vi "Parse Algorithm Inputs.vi"(8 "error in (no error)":errorcluster, 11 "Algorithm Information":T2) -> (0 "error out":errorcluster, 1 "Required Q as string":string, 2 "Optional Q as string":string, 3 "Groups of Alternatives":cluster{T1[], "is Optional?":bool}[](array[cluster]), 4 "Q descriptions":string)   [LabVIEW 2013, in "QWTBLVLib.lvlib"]
doc: "Returns parsed informations about required, alternative and parameter input quantities."
uses:
  QWTBLVLib.lvlib
  TD Algorithm Information.ctl
  TD Algorithm Information Input.ctl
  TD Algorithm Information Output.ctl
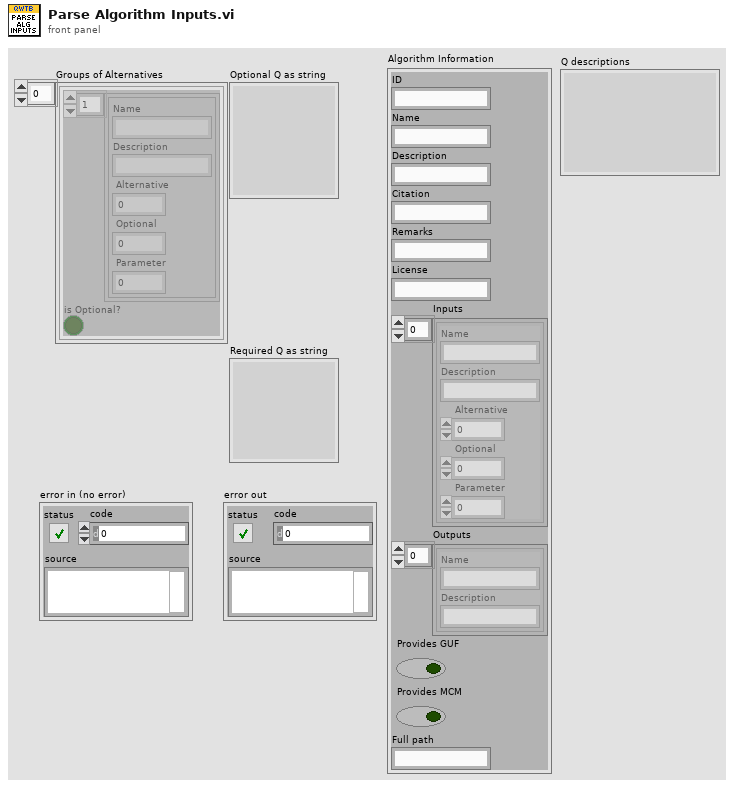
[diagram p1: front panel]
types:
  T1 = typedef "QWTBLVLib.lvlib/TD Algorithm Information Input.ctl" = cluster{"Name":string, "Description":string, "Alternative":i32, "Optional":i32, "Parameter":i32}
  T2 = typedef "QWTBLVLib.lvlib/TD Algorithm Information.ctl" = cluster{"ID":string, "Name":string, "Description":string, "Citation":string, "Remarks":string, "License":string, "Inputs":T1[], "Outputs":T3[], "Provides GUF":bool, "Provides MCM":bool, "Full path":string}
  T3 = typedef "QWTBLVLib.lvlib/TD Algorithm Information Output.ctl" = cluster{"Name":string, "Description":string}
  T4 = cluster{"Group of Alternatives":T1[], "is Group Optional?":bool}[]
  T5 = cluster{"Group of Alternatives":T1[], "is Group Optional?":bool}
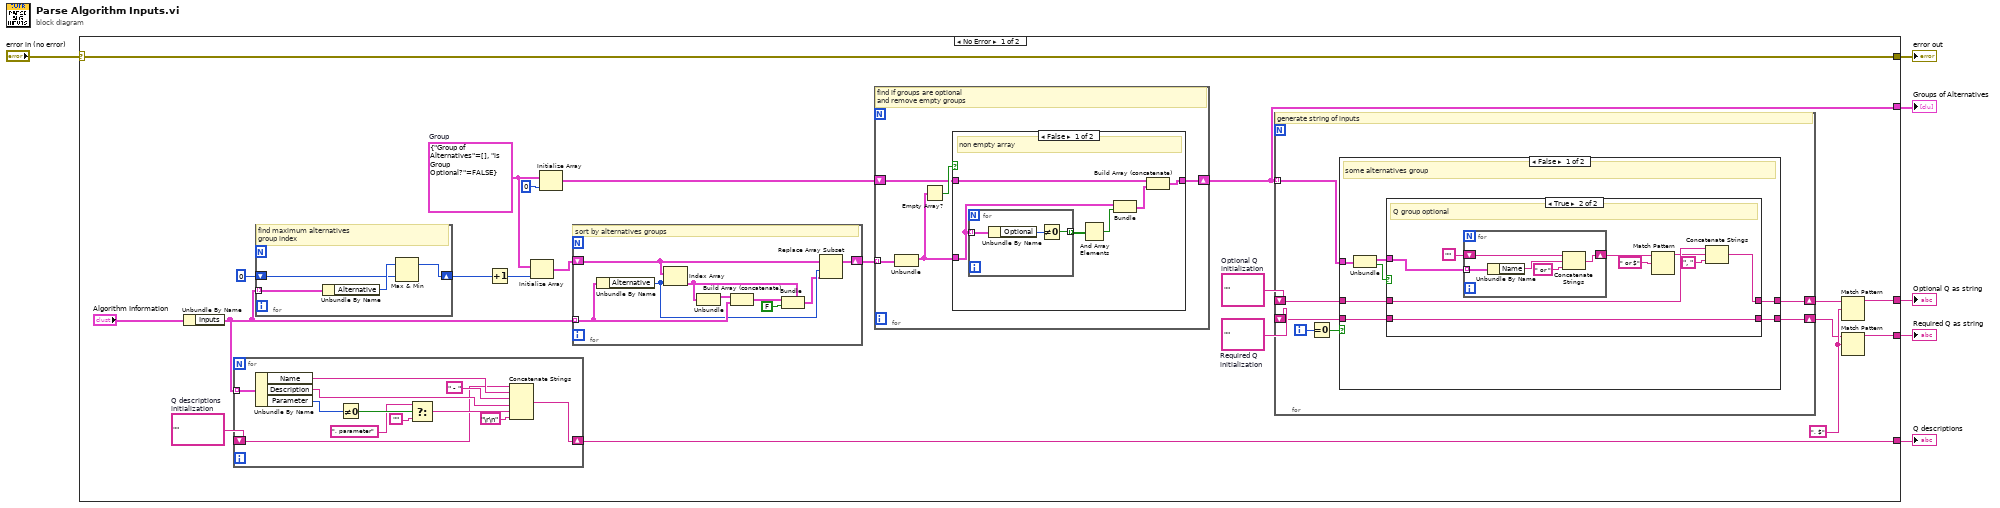
[diagram p0: block diagram]
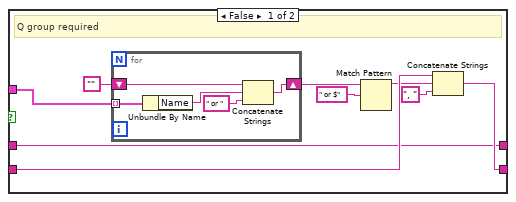
[diagram p2: hidden frame]
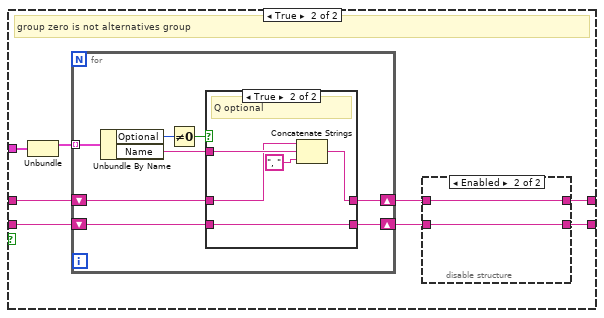
[diagram p3: hidden frame]
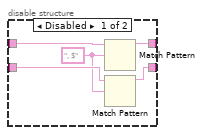
[diagram p4: hidden frame]
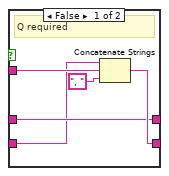
[diagram p5: hidden frame]
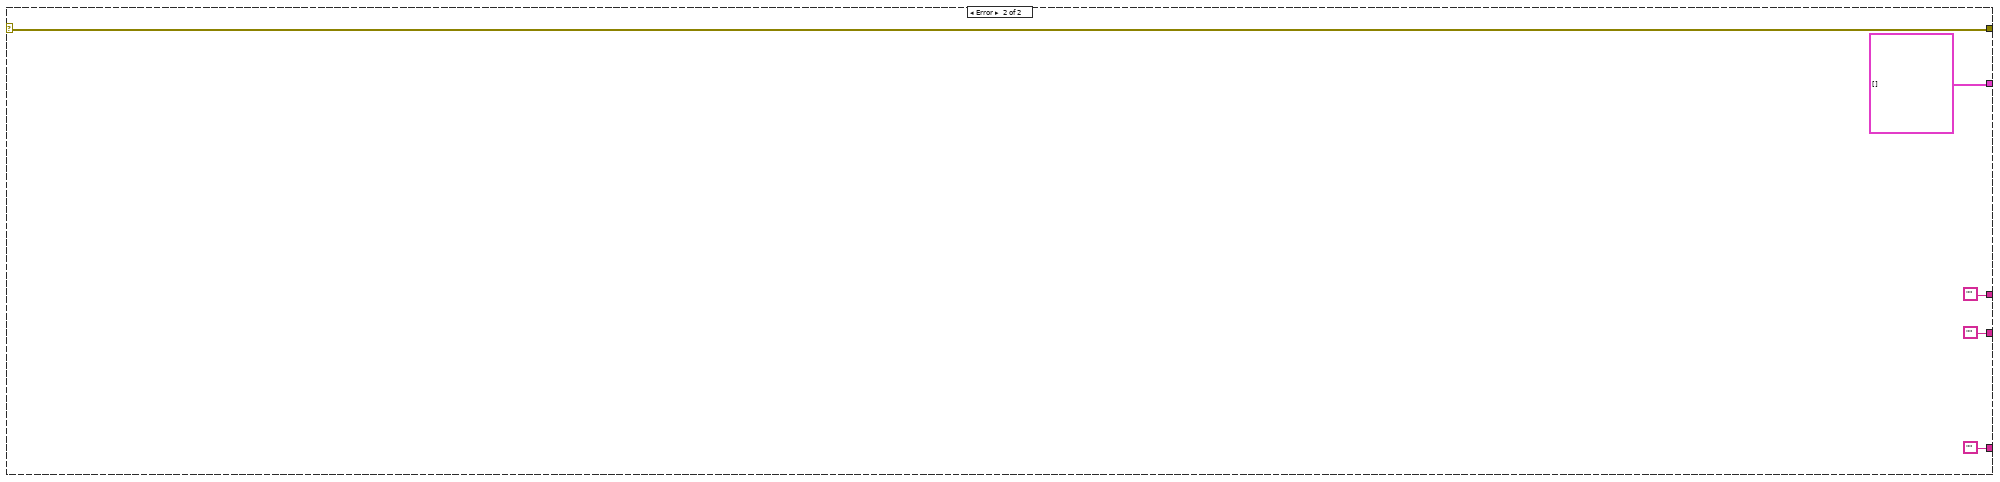
[diagram p7: hidden frame]
diagram:
  n1 = case shown="No Error" "error in (no error)" {
    selector: "error in (no error)" -> [w26 w147]
    tunnel: [w26 w147] -> w6
    tunnel: [w12 T4 []] -> w4
    tunnel: [w9 ""] -> w3
    tunnel: [w8 ""] -> w2
    tunnel: [w7 ""] -> w1
    frame No Error {
      w10 = ""  # Q descriptions initialization
      w15 = ", $" ("regular expression")
      w22 = ""  # Optional Q initialization
      w23 = ""  # Required Q initialization
      w18 = T5 {"Group of Alternatives"=[], "is Group Optional?"=FALSE}  # Group
      n2 = Unbundle By Name("Algorithm Information") -> ("Inputs"=w11:T1[])
      n3 = for {
        tunnel: w11 -> [w39] mode=indexing
        shift-right: [w29] -> w7
        shift-left: w10 -> [w28]
        n4 = Unbundle By Name(w39) -> ("Name"=w34:string, "Description"=w33:string, "Parameter"=w38:i32)
        n5 = Not Equal To 0?(x=w38) -> (x != 0?=w37:bool)
        n6 = Select(t=", parameter" ("format string"), s=w37, f="") -> (s? t:f=w32:string)
        n7 = Concatenate Strings(w28, w34, " - " ("string"), w33, w32, "\r\n") -> (w29:string)
      }
      n8 = for {
        tunnel: w11 -> [w118] mode=indexing
        shift-right: [w115] -> w21
        shift-left: 0 ("Alternative") -> [w116]
        # "find maximum alternatives\ngroup index"
        n9 = Unbundle By Name(w118) -> ("Alternative"=w117:i32)
        n10 = Max & Min(x=w117, y=w116) -> (max(x,y)=w115:i32)  [unwired: 1 out]
      }
      n11 = Increment(x=w21) -> (x+1=w20:i32)
      n12 = Initialize Array(w18, w20) -> (w24:T4)
      n13 = Initialize Array(w18, 0 ("dimension size")) -> (w16:T4)
      n14 = for {
        tunnel: w11 -> [w142] mode=indexing
        shift-right: [w136] -> w19
        shift-left: w24 -> [w135]
        # "sort by alternatives groups"
        n15 = Unbundle By Name(w142) -> ("Alternative"=w138:i32)
        n16 = Index Array(array=w135, index=w138) -> (element=w139:T5)
        n17 = Unbundle(w139) -> ("Group of Alternatives"=w140:T1[])  [unwired: 1 out]
        n18 = Build Array (concatenate)(w140, w142) -> (w141:T1[])
        n19 = Bundle(cluster=w139, "Group of Alternatives"=w141, "is Group Optional?"=FALSE) -> (w137:T5)
        n20 = Replace Array Subset(array=w135, new element=w137, index=w138) -> (w136:T4)
      }
      n21 = for {
        tunnel: w19 -> [w123] mode=indexing
        shift-right: [w119] -> w12
        shift-left: w16 -> [w120]
        # "find if groups are optional\nand remove empty groups"
        n22 = Unbundle(w123) -> ("Group of Alternatives"=w122:T1[])  [unwired: 1 out]
        n23 = Empty Array?(array=w122) -> (empty?=w121:bool)
        n24 = case shown="False" w121 {
          tunnel: w122 -> [w127 _]
          tunnel: w120 -> [w125 w133]
          tunnel: [w124 w133] -> w119
          frame False {
            # "non empty array"
            n25 = for {
              tunnel: w127 -> [w132] mode=indexing
              tunnel: [w130] -> w128 mode=indexing
              n26 = Unbundle By Name(w132) -> ("Optional"=w131:i32)
              n27 = Not Equal To 0?(x=w131) -> (x != 0?=w130:bool)
            }
            n28 = And Array Elements(Boolean array=w128) -> (logical AND=w129:bool)
            n29 = Bundle("Group of Alternatives"=w127, w129) -> (w126:cluster{"Group of Alternatives":T1[], bool})  [unwired: 1 in]
            n30 = Build Array (concatenate)(w125, w126) -> (w124:T4)
          }
          frame True {
            # "empty array"
          }
        }
      }
      n31 = for {
        tunnel: w12 -> [w44] mode=indexing
        shift-right: [w42] -> w14
        shift-left: w22 -> [w40]
        shift-right: [w41] -> w13
        shift-left: w23 -> [w43]
        i -> [w46]
        # "generate string of inputs"
        n32 = Equal To 0?(x=w46) -> (x = 0?=w45:bool)
        n33 = case shown="False" w45 {
          tunnel: w44 -> [w53 w89]
          tunnel: w43 -> [w48 w87]
          tunnel: [w49 w84] -> w42
          tunnel: [w47 w82] -> w41
          tunnel: w40 -> [w50 w86]
          frame False {
            # "some alternatives group"
            n34 = Unbundle(w53) -> ("Group of Alternatives"=w51:T1[], "is Group Optional?"=w52:bool)
            n35 = case shown="True" w52 {
              tunnel: w51 -> [w60 w76]
              tunnel: w50 -> [w57 w74]
              tunnel: [w57 w72] -> w49
              tunnel: w48 -> [w59 w71]
              tunnel: [w58 w71] -> w47
              frame False {
                # "Q group required"
                n36 = for {
                  tunnel: w60 -> [w66] mode=indexing
                  shift-right: [w63] -> w55
                  shift-left: "" -> [w67]
                  n37 = Unbundle By Name(w66) -> ("Name"=w65:string)
                  n38 = Concatenate Strings(w67, w65, " or " ("string")) -> (w63:string)
                }
                n39 = Match Pattern(string=w55, regular expression=" or $") -> (before substring=w54:string)  [unwired: 1 in, 3 out]
                n40 = Concatenate Strings(w59, w54, ", " ("string")) -> (w58:string)
              }
              frame True {
                # "Q group optional"
                n41 = for {
                  tunnel: w76 -> [w80] mode=indexing
                  shift-right: [w77] -> w69
                  shift-left: "" -> [w81]
                  n42 = Unbundle By Name(w80) -> ("Name"=w79:string)
                  n43 = Concatenate Strings(w81, w79, " or " ("string")) -> (w77:string)
                }
                n44 = Match Pattern(string=w69, regular expression=" or $") -> (before substring=w68:string)  [unwired: 1 in, 3 out]
                n45 = Concatenate Strings(w74, w68, ", " ("string")) -> (w72:string)
              }
            }
          }
          frame True {
            # "group zero is not alternatives group"
            n46 = Unbundle(w89) -> ("Group of Alternatives"=w88:T1[])  [unwired: 1 out]
            n47 = for {
              tunnel: w88 -> [w104] mode=indexing
              shift-right: [w99] -> w85
              shift-left: w86 -> [w97]
              shift-right: [w98] -> w83
              shift-left: w87 -> [w100]
              n48 = Unbundle By Name(w104) -> ("Optional"=w103:i32, "Name"=w101:string)
              n49 = Not Equal To 0?(x=w103) -> (x != 0?=w102:bool)
              n50 = case shown="True" w102 {
                tunnel: w101 -> [w109 w113]
                tunnel: w100 -> [w105 w111]
                tunnel: [w106 w114] -> w99
                tunnel: [w108 w111] -> w98
                tunnel: w97 -> [w106 w110]
                frame False {
                  # "Q required"
                  n51 = Concatenate Strings(w105, w109, ", " ("string")) -> (w108:string)
                }
                frame True {
                  # "Q optional"
                  n52 = Concatenate Strings(w110, w113, ", " ("string")) -> (w114:string)
                }
              }
            }
            n53 = disable-structure shown="Enabled" {
              disable-tunnel: w85 -> [w94 w95]
              disable-tunnel: [w93 w95] -> w84
              disable-tunnel: w83 -> [w92 w96]
              disable-tunnel: [w91 w96] -> w82
              frame Disabled {
                w90 = ", $" ("regular expression")
                n54 = Match Pattern(string=w94, regular expression=w90) -> (before substring=w93:string)  [unwired: 1 in, 3 out]
                n55 = Match Pattern(string=w92, regular expression=w90) -> (before substring=w91:string)  [unwired: 1 in, 3 out]
              }
              frame Enabled {
              }
            }
          }
        }
      }
      n56 = Match Pattern(string=w14, regular expression=w15) -> (before substring=w8:string)  [unwired: 1 in, 3 out]
      n57 = Match Pattern(string=w13, regular expression=w15) -> (before substring=w9:string)  [unwired: 1 in, 3 out]
    }
    frame Error {
    }
  }
  "error out" <- w6
  "Groups of Alternatives" <- w4
  "Optional Q as string" <- w2
  "Required Q as string" <- w3
  "Q descriptions" <- w1
